vi "Create Data Channel - Array - Format.vi"(8 "Error In":errorcluster, 9 "Settings":T2, 10 "Name":string, 11 "Message Refnum In":T1 format="%.0x") -> (0 "Error Out":errorcluster, 2 "Channel Refnums":T1[](array[typedef]) format="%.0x", 3 "Message Refnum Out":T1 format="%.0x")   [LabVIEW 2018, in "Instrument Addon Scripting API.lvlib"]
doc: "Creates a new Data Array with the following configuration: \nData Type: Array\nChannel Type: Format\n\nIt also adds all the channels to the Data Array specified in the \"Settings\".\n\nInput: \nMessage Refnum In: reference to the \"Response\" message section.\nName: represents the desired name of the Data Array.\nSettings: represents the settings applied on the Data Array, as well as the Data Channels which will be added to the Data Array (Name, Default Value, Units).\n\nOutput:\nMessage Refnum Out: reference to the \"Response\" message section used as input.\nChannel Renum: reference to the newly created Data Array section."
uses:
  Instrument Addon Scripting API.lvlib
  <vilib>/NI Veristand/Custom Device API/Custom Device Item Ref.ctl
  TypeDefs/Array Format Settings.ctl
  TypeDefs/Array Element.ctl
  Addon/Addon Shared/Types/Data Parameters.ctl
  Addon/Addon Shared/Types/Protocol Data Type.ctl
  Addon/Addon Shared/Types/Data Channel Type.ctl
  Addon/Addon Shared/Types/Type Cast Type.ctl
  Addon/Addon Shared/Types/Endian.ctl
  Addon/Addon Shared/Instrument Addon Shared.lvlib
  <vilib>/NI Veristand/Custom Device API/Custom Device API.lvlib
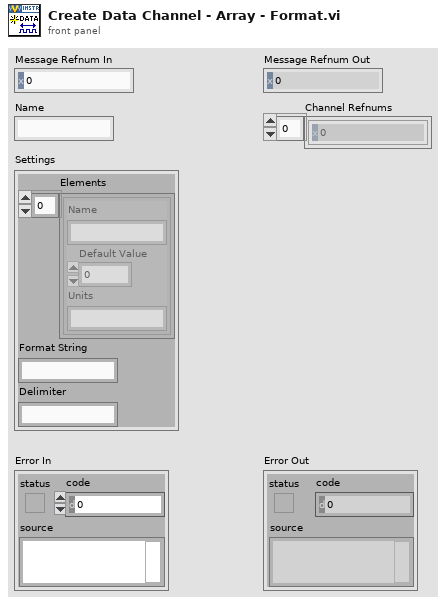
[diagram p1: front panel]
types:
  T1 = typedef "Custom Device API.lvlib/Custom Device Item Ref.ctl" = u64
  T2 = typedef "Instrument Addon Scripting API.lvlib/Array Format Settings.ctl" = cluster{"Elements":T3[], "Format String":string, "Delimiter":string}
  T3 = typedef "Instrument Addon Scripting API.lvlib/Array Element.ctl" = cluster{"Name":string, "Default Value":dbl, "Units":string}
  T4 = typedef "Instrument Addon Shared.lvlib/Data Channel Type.ctl" = enum16{"Format", "Comparison", "Type Cast", "Enumerated List"}
  T5 = typedef "Instrument Addon Shared.lvlib/Protocol Data Type.ctl" = enum16{"Single Channel", "Array"}
  T6 = typedef "Instrument Addon Shared.lvlib/Data Parameters.ctl" = cluster{"Data Type":T5, "Channel Type":T4, "Format String":string, "Expected String":string, "Type":T7, "List":string[], "Delimiter":string, "Endian":T8}
  T7 = typedef "Instrument Addon Shared.lvlib/Type Cast Type.ctl" = enum16{"DBL", "SGL", "U64", "U32", "U16", "U8", "I64", "I32", "I16", "I8"}
  T8 = typedef "Instrument Addon Shared.lvlib/Endian.ctl" = enum16{"Native", "Little", "Big"}
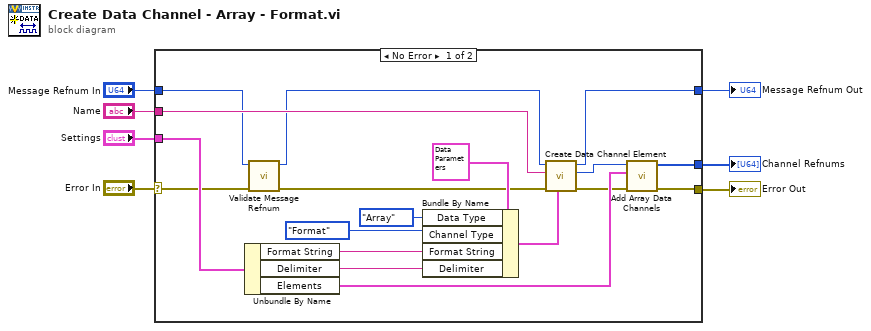
[diagram p0: block diagram]
diagram:
  n1 = case shown="No Error" "Error In" {
    selector: "Error In" -> [w11 w27]
    tunnel: [w20 w27] -> w7
    tunnel: [w14 w26] -> w6
    tunnel: "Name" -> [w16 _]
    tunnel: "Message Refnum In" -> [w9 w26]
    tunnel: "Settings" -> [w19 _]
    tunnel: [w18 _] -> w1
    frame No Error {
      n2 = Unbundle By Name(w19) -> ("Format String"=w22:string, "Delimiter"=w21:string, "Elements"=w17:T3[])
      n3 = call "Validate Message Refnum.vi"("error in (no error)"=w11, "Message in"=w9) -> ("error out"=w10:errorcluster, "Message out"=w8:T1)  [unwired: 8 in]
      n4 = Bundle By Name(cluster=T6 {"Data Type"=enum."Array", "Channel Type"=enum."Format", "Format String"="%.3g", "Expected String"="", "Type"=enum."SGL", "List"=[], "Delimiter"=",", "Endian"=enum."Native"} ("Settings"), "Data Type"=Protocol_Data_Type."Array", "Channel Type"=Data_Channel_Type."Format", "Format String"=w22, "Delimiter"=w21) -> (w15:T6)
      n5 = call "Create Data Channel Element.vi"("Data Channel Parameters"=w15, "Error In"=w10, "Name"=w16, "Refnum In"=w8) -> ("Error Out"=w12:errorcluster, "Channel Refnum"=w13:T1, "Refnum Out"=w14:T1)  [unwired: 5 in]
      n6 = call "Add Array Data Channels.vi"("Error In"=w12, "Array Elements"=w17, "Section Refnum In"=w13) -> ("Error Out"=w20:errorcluster, "Channel Refnums"=w18:T1[])  [unwired: 7 in]
    }
    frame Error {
    }
  }
  "Error Out" <- w7
  "Message Refnum Out" <- w6
  "Channel Refnums" <- w1
